vi "Initialize Target Config.vi"(8 "error in (no error)":errorcluster, 11 "Console Ref In":refnum<vi>) -> (0 "error out":errorcluster, 3 "Console Ref Out":refnum<vi>)   [LabVIEW 2015]
doc: "Do all initialization necessary for target configuration."
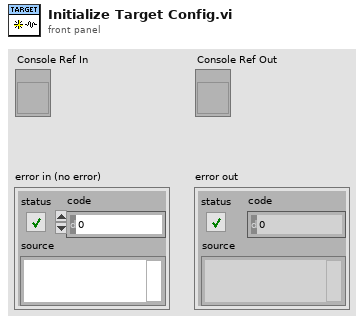
[diagram p1: front panel]
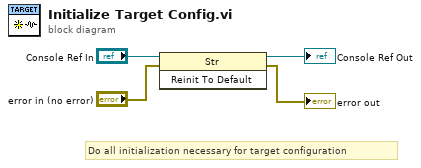
[diagram p0: block diagram]
diagram:
  # "Do all initialization necessary for target configuration"
  n1 = invoke class="Str" method="Reinit To Default"(reference="Console Ref In", error in="error in (no error)") -> (reference out=→"Console Ref Out":refnum<vi>, error out=→"error out":errorcluster)  [unwired: 1 in, 1 out]
